vi "CRYLimit Curves Name Replace.vi"(6 "StepName":string, 7 "Setup in":T1={"No.VI"=0, "Category"="", "StepName"="", "Seq setup flattened"="", "Comment"="", "Steps config."=[], "Jump config"=[], "Start"=0.0, "Increment"=0.0, "Name"="Pa", "Unit"="Pa", "Y data"=1, "Y prefix"="", "Y dB ref"=1.0, "Y unit"="", "Repeat State Array"=[]} {"Repeat State Array"."Start" format="%#_5g"; "Y dB ref" format="%.1f"; "Y data" items=["dB", "Lin"]; "Start" format="%#_5g"}, 8 "Hardware Setup In":string, 9 "Step Set up In":string, 11 "Type In":string) -> (3 "Inserted Names Out":string[](array[string]))   [LabVIEW 2013]
uses:
  Typedef Control/CRYStep.ctl
  Typedef Control/CRYData Cluster.ctl
  Typedef Control/CRYWaveform Cluster.ctl
  Typedef Control/CRYResult Cluster.ctl
  CRYMainGlobal.vi
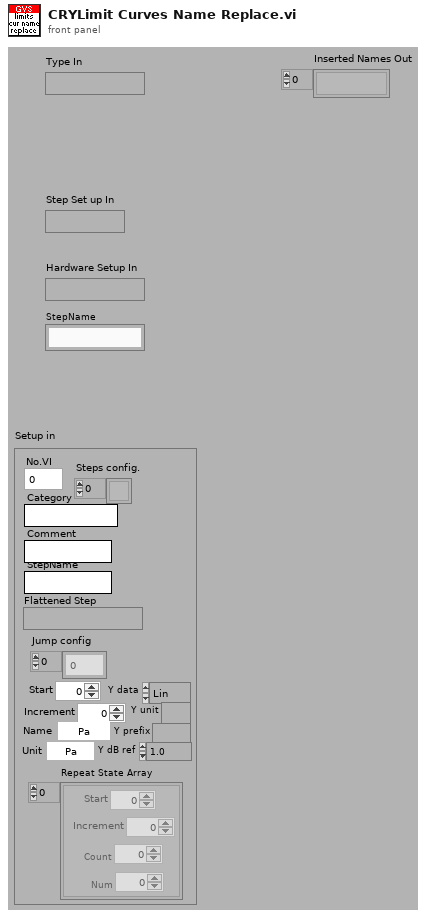
[diagram p1: front panel]
types:
  T1 = typedef "CRYStep.ctl" = cluster{"No.VI":i32, "Category":string, "StepName":string, "Seq setup flattened":string, "Comment":string, "Steps config.":bool[], "Jump config":i32[], "Start":dbl, "Increment":dbl, "Name":string, "Unit":string, "Y data":u16, "Y prefix":string, "Y dB ref":dbl, "Y unit":string, "Repeat State Array":cluster{"Start":dbl, "Increment":dbl, "Count":i32, "Num":i32}[]}
  T2 = typedef "CRYResult Cluster.ctl" = cluster{"Name":string, "Margin":dbl, "unit":string, "Verdict":bool, "Limit":string, "Max/Min":string, "protected":bool, "Step No.":i32, "Test Info":string, "AutoProtect":bool}
  T3 = typedef "CRYWaveform Cluster.ctl" = cluster{"Waveform":cluster{"X0":dbl, "dX":dbl, "Y":sgl[]}, "X data":u16, "Y data":u16, "Y axis":u16, "X unit":string, "Y unit":string, "Y dB ref":dbl, "display Y":bool, "display X":bool, "Overload?":bool, "Test Info":string, "Step No.":i32, "Name":string, "protected":bool, "Sqc history":string[], "Signal Channel ID":i32, "Plot Settings":cluster{"Color":u32, "Interpolation":u8, "Point Style":u8, "Line Style":u8, "Point Color":u32, "Line Width":u8, "Bar Plot Style":u8, "Fill To":i16}, "AutoProtect":bool}
  T4 = typedef "CRYData Cluster.ctl" = cluster{"Name":string, "Curve":cluster{"x":dbl, "y":dbl, "z":dbl}[], "X data":u16, "Y data":u16, "Z data":u16, "X axis":u16, "Y axis":u16, "Z axis":u16, "X unit":string, "Y unit":string, "Z unit":string, "X dB ref":dbl, "Y dB ref":dbl, "Z dB ref":dbl, "single val":bool, "protected":bool, "display X":bool, "display Y":bool, "display Z":bool, "Test Info":string, "Step No.":i32, "Plot Settings":cluster{"Color":u32, "Interpolation":u8, "Point Style":u8, "Line Style":u8, "Point Color":u32, "Line Width":u8, "Bar Plot Style":u8, "Fill To":i16}, "AutoProtect":bool}
  T5 = typedef "CRYLimits.ctl" = cluster{"Name":string, "Tolerance":u16, "X Axis":u16, "Limits":u16, "Upper Limit":cluster{dbl, dbl}[], "Align Ref":cluster{dbl, dbl}, "Lower Limit":cluster{dbl, dbl}[], "Y data":u16, "Y unit":string, "Y dB ref":dbl, "Curve Names":string[], "Y-Resolution":u8, "Type":u16, "x float":bool, "X min-max-step":cluster{"Limit X Offset Min":dbl, "Limit X Offset Max":dbl, "Limit X Offset Step Size":dbl}, "magn/phase":u16, "Upper Limit Type":u16, "Lower Limit Type":u16, "Lim Curve axis up":u16, "Lim Curve axis lo":u16, "Data Selection Upper":u16, "Data Selection Lower":u16, "X-Resolution":u8, "Output failed point curves?":bool, "X data":u16, "X unit":string, "X dB ref":dbl, "X-Y Graph Set-up":string, "Tab Value":enum32{"Data", "Parameters"}, "Help":string, "X Up Val":dbl, "Y Up Val":dbl, "X Low Val":dbl, "Y Low Val":dbl, "Up Limit Val":dbl, "Low Limit Val":dbl, "bAdd DataName":bool, "Custom Name":string}
  T6 = cluster{"Start":dbl, "Increment":dbl, "Count":i32, "Num":i32}[]
  T7 = enum32{"English", "Chinese", "Korean", "Japanese", "Russian", "Chinese traditional"}
  T8 = typedef "CRYData Cluster Array.ctl" = T4[]
  T9 = typedef "CRYWaveform Cluster Array.ctl" = T3[]
  T10 = typedef "CRYResult Cluster Array.ctl" = T2[]
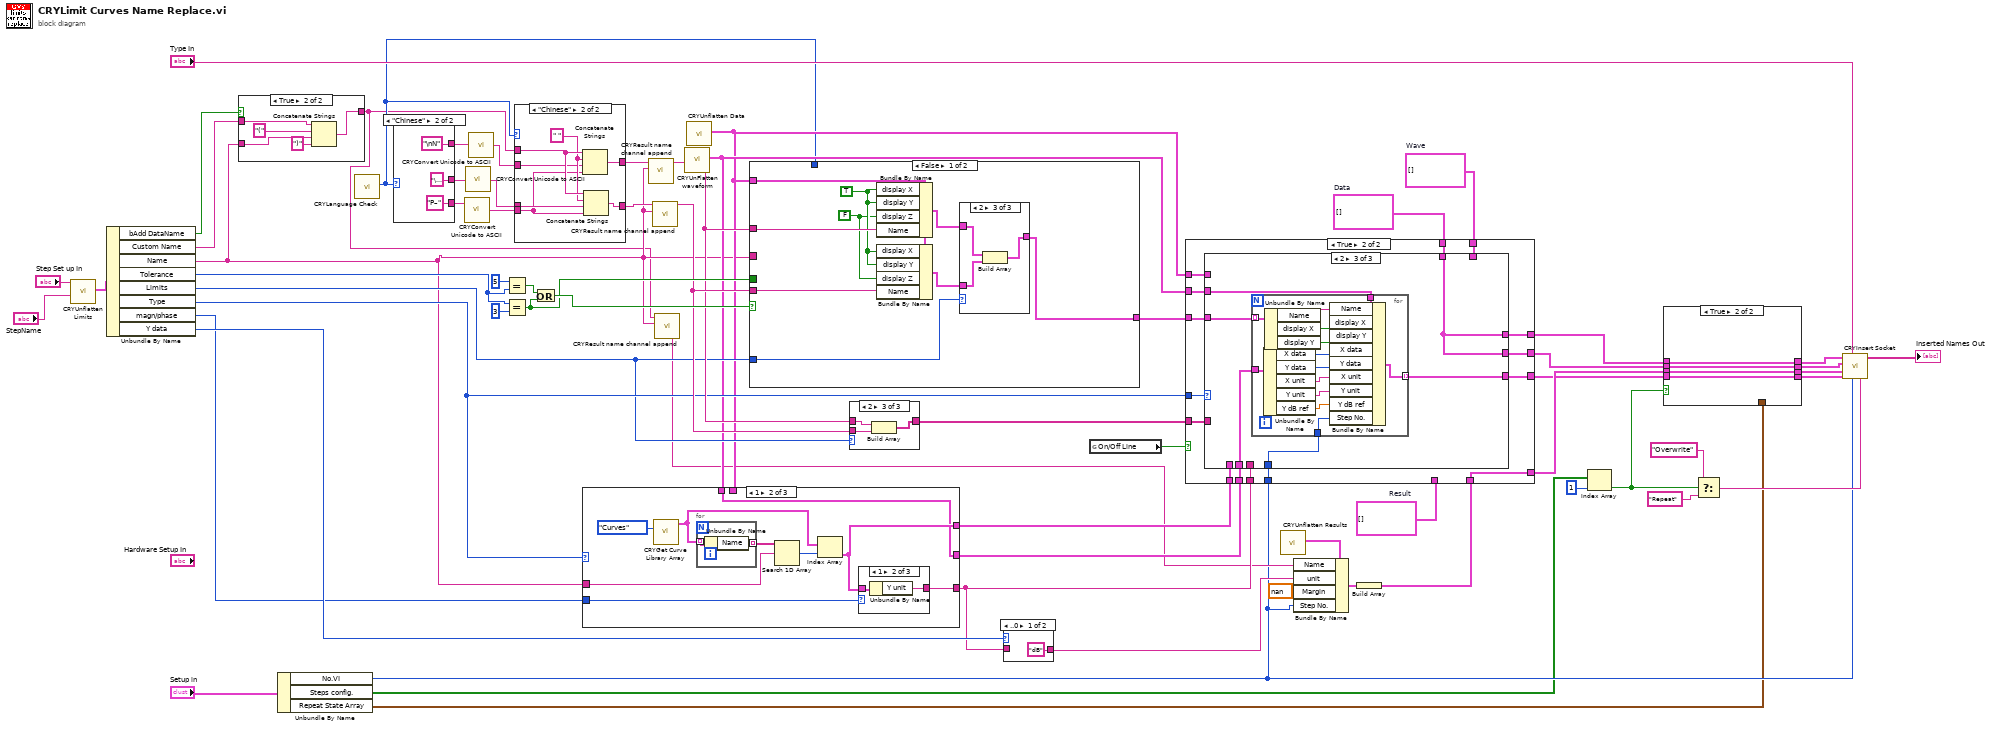
[diagram p0: block diagram]
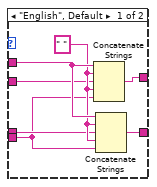
[diagram p3: hidden frame]
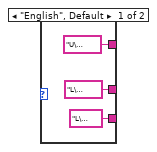
[diagram p4: hidden frame]
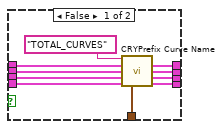
[diagram p5: hidden frame]
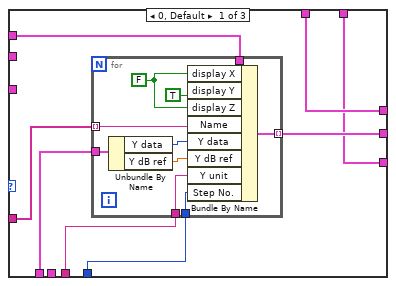
[diagram p7: hidden frame]
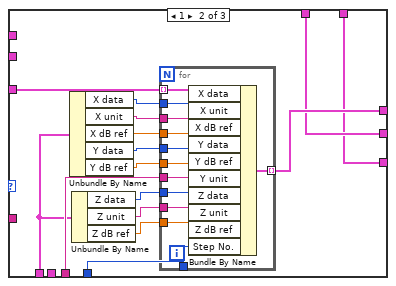
[diagram p8: hidden frame]
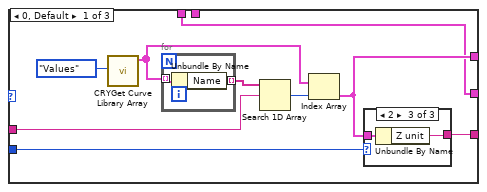
[diagram p9: hidden frame]
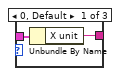
[diagram p10: hidden frame]
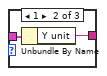
[diagram p11: hidden frame]
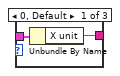
[diagram p12: hidden frame]
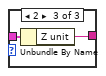
[diagram p13: hidden frame]
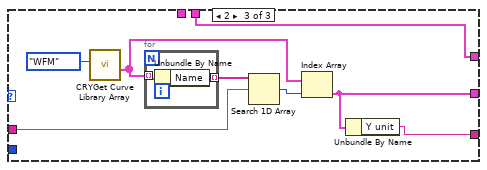
[diagram p14: hidden frame]
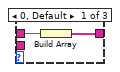
[diagram p16: hidden frame]
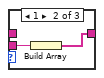
[diagram p17: hidden frame]
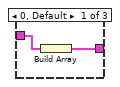
[diagram p18: hidden frame]
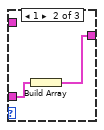
[diagram p19: hidden frame]
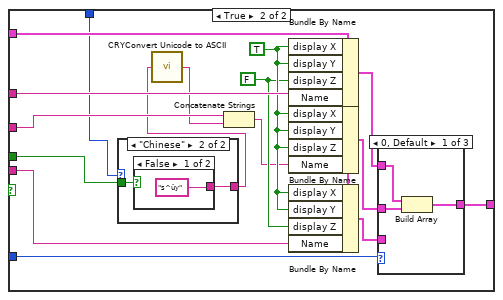
[diagram p20: hidden frame]
diagram:
  w31 = T2[] []  # Result
  w34 = T3[] []  # Wave
  w35 = T4[] []  # Data
  n1 = call "CRYUnflatten Limits.vi"("Step Name"="StepName", "Unflatten Limits"="Step Set up In") -> ("Limits"=w45:T5)  [unwired: 7 in, 2 out]
  n2 = Unbundle By Name(w45) -> ("bAdd DataName"=w5:bool, "Custom Name"=w4:string, "Name"=w3:string, "Tolerance"=w58:u16, "Limits"=w39:u16, "Type"=w44:u16, "magn/phase"=w43:u16, "Y data"=w52:u16)
  n3 = case shown="True" w5 {
    tunnel: w4 -> [w65 w70]
    tunnel: w3 -> [_ w68]
    tunnel: [w65 w66] -> w2
    frame False {
    }
    frame True {
      n4 = Concatenate Strings(w70, "(" ("string"), w68, ")" ("string")) -> (w66:string)
    }
  }
  n5 = Unbundle By Name("Setup in") -> ("No.VI"=w24:i32, "Steps config."=w23:bool[], "Repeat State Array"=w13:T6)
  n6 = call "CRYLanguage Check.vi"() -> ("Language"=w6:T7)  [unwired: 10 in, 1 out]
  n7 = case shown="\"Chinese\"" w6 {
    tunnel: ["L\u0000o\u0000w\u0000e\u0000r\u0000" ("Name") "\u000bN" ("Name")] -> w12
    tunnel: ["L\u0000i\u0000m\u0000i\u0000t\u0000" ("Name") "P–" ("Name")] -> w11
    tunnel: ["U\u0000p\u0000p\u0000e\u0000r\u0000" ("Name") "\nN" ("Name")] -> w10
    frame "English", Default {
    }
    frame "Chinese" {
    }
  }
  n8 = call "CRYConvert Unicode to ASCII.vi"("Unicode"=w11) -> ("ASCII"=w7:string)  [unwired: 4 in]
  n9 = call "CRYConvert Unicode to ASCII.vi"("Unicode"=w12) -> ("ASCII"=w8:string)  [unwired: 4 in]
  n10 = call "CRYConvert Unicode to ASCII.vi"("Unicode"=w10) -> ("ASCII"=w9:string)  [unwired: 4 in]
  n11 = Equal?(x=u16 5, y=w58) -> (x = y?=w59:bool)
  n12 = Equal?(x=w58, y=u16 3) -> (x = y?=w56:bool)
  n13 = case shown="\"Chinese\"" w6 {
    tunnel: [w83 w90] -> w63
    tunnel: [w82 w89] -> w62
    tunnel: w2 -> [w81 w88]
    tunnel: w9 -> [w79 w86]
    tunnel: w8 -> [w78 w85]
    tunnel: w7 -> [w77 w84]
    frame "English", Default {
      w80 = " " ("Name")
      n14 = Concatenate Strings(w81, w80, w79, w80, w77) -> (w83:string)
      n15 = Concatenate Strings(w81, w80, w78, w80, w77) -> (w82:string)
    }
    frame "Chinese" {
      w87 = " " ("Name")
      n16 = Concatenate Strings(w88, w87, w86, w84) -> (w90:string)
      n17 = Concatenate Strings(w88, w87, w85, w84) -> (w89:string)
    }
  }
  n18 = Or(x=w59, y=w56) -> (x .or. y?=w57:bool)
  n19 = call "CRYResult name channel append.vi"("Curve selected"=w3, "Limit step name (no ext.)"=w63) -> ("Result name with channel suffix"=w49:string)  [unwired: 9 out]
  n20 = call "CRYResult name channel append.vi"("Curve selected"=w3, "Limit step name (no ext.)"=w62) -> ("Result name with channel suffix"=w55:string)  [unwired: 9 out]
  n21 = call "CRYResult name channel append.vi"("Curve selected"=w3, "Limit step name (no ext.)"=w2) -> ("Result name with channel suffix"=w30:string)  [unwired: 9 out]
  n22 = call "CRYUnFlatten waveform.vi"() -> ("Waveform Cluster"=w38:T3)  [unwired: 9 in, 2 out]
  n23 = call "CRYUnflatten Data.vi"() -> ("Datum"=w37:T4)  [unwired: 9 in, 2 out]
  n24 = case shown="1" w44 {
    tunnel: w3 -> [w97 w114 w130]
    tunnel: [w94 w110 w125] -> w41
    tunnel: w43 -> [w93 w111 _]
    tunnel: [w92 w109 w127] -> w42
    tunnel: [w91 w108 w126] -> w40
    tunnel: w38 -> [w91 w108 _]
    tunnel: w37 -> [_ _ w125]
    frame 0, Default {
      n25 = call "CRYGet Curve Library Array.vi"("Type In"=enum16{"Curves", "Values", "Results", "WFM"}."Values" ("Type")) -> ("Curve/Value array"=w95:T8)  [unwired: 10 out]
      n26 = for {
        tunnel: w95 -> [w107] mode=indexing
        tunnel: [w106] -> w98 mode=indexing
        n27 = Unbundle By Name(w107) -> ("Name"=w106:string)
      }
      n28 = Search 1D Array(1D array=w98, element=w97) -> (index of element=w96:i32)  [unwired: 1 in]
      n29 = Index Array(array=w95, index=w96) -> (element=w94:T4)
      n30 = case shown="2" w93 {
        tunnel: w94 -> [w101 w103 w105]
        tunnel: [w100 w102 w104] -> w92
        frame 0, Default {
          n31 = Unbundle By Name(w101) -> ("X unit"=w100:string)
        }
        frame 1 {
          n32 = Unbundle By Name(w103) -> ("Y unit"=w102:string)
        }
        frame 2 {
          n33 = Unbundle By Name(w105) -> ("Z unit"=w104:string)
        }
      }
    }
    frame 1 {
      n34 = call "CRYGet Curve Library Array.vi"("Type In"=enum16{"Curves", "Values", "Results", "WFM"}."Curves" ("Type")) -> ("Curve/Value array"=w112:T8)  [unwired: 10 out]
      n35 = for {
        tunnel: w112 -> [w124] mode=indexing
        tunnel: [w123] -> w115 mode=indexing
        n36 = Unbundle By Name(w124) -> ("Name"=w123:string)
      }
      n37 = Search 1D Array(1D array=w115, element=w114) -> (index of element=w113:i32)  [unwired: 1 in]
      n38 = Index Array(array=w112, index=w113) -> (element=w110:T4)
      n39 = case shown="1" w111 {
        tunnel: w110 -> [w118 w120 w122]
        tunnel: [w117 w119 w121] -> w109
        frame 0, Default {
          n40 = Unbundle By Name(w118) -> ("X unit"=w117:string)
        }
        frame 1 {
          n41 = Unbundle By Name(w120) -> ("Y unit"=w119:string)
        }
        frame 2 {
          n42 = Unbundle By Name(w122) -> ("Z unit"=w121:string)
        }
      }
    }
    frame 2 {
      n43 = call "CRYGet Curve Library Array.vi"("Type In"=enum16{"Curves", "Values", "Results", "WFM"}."WFM" ("Type")) -> ("Waveform Array"=w128:T9)  [unwired: 10 out]
      n44 = for {
        tunnel: w128 -> [w134] mode=indexing
        tunnel: [w133] -> w131 mode=indexing
        n45 = Unbundle By Name(w134) -> ("Name"=w133:string)
      }
      n46 = Search 1D Array(1D array=w131, element=w130) -> (index of element=w129:i32)  [unwired: 1 in]
      n47 = Index Array(array=w128, index=w129) -> (element=w126:T3)
      n48 = Unbundle By Name(w126) -> ("Y unit"=w127:string)
    }
  }
  n49 = case shown="False" w57 {
    tunnel: w56 -> [_ w166]
    tunnel: w49 -> [w141 w164]
    tunnel: w55 -> [w139 w161]
    tunnel: w39 -> [w143 w165]
    tunnel: [w142 w158] -> w53
    tunnel: w37 -> [w140 w160]
    tunnel: w3 -> [_ w155]
    tunnel: w6 -> [_ w151]
    frame False {
      w135 = FALSE ("display Z")
      w136 = TRUE ("display X")
      n50 = Bundle By Name(cluster=w140, "display X"=w136, "display Y"=w136, "display Z"=w135, "Name"=w141) -> (w138:T4)
      n51 = Bundle By Name(cluster=w140, "display X"=w136, "display Y"=w136, "display Z"=w135, "Name"=w139) -> (w137:T4)
      n52 = case shown="2" w143 {
        tunnel: w138 -> [w145 _ w150]
        tunnel: w137 -> [_ w147 w149]
        tunnel: [w144 w146 w148] -> w142
        frame 0, Default {
          n53 = Build Array(w145) -> (w144:T4[])
        }
        frame 1 {
          n54 = Build Array(w147) -> (w146:T4[])
        }
        frame 2 {
          n55 = Build Array(w150, w149) -> (w148:T4[])
        }
      }
    }
    frame True {
      w156 = FALSE ("display Z")
      w157 = TRUE ("display X")
      n56 = case shown="\"Chinese\"" w151 {
        tunnel: w166 -> [w168 w172]
        tunnel: [w167 w171] -> w153
        frame "English", Default {
          n57 = case shown="True" w168 {
            tunnel: [" \u0000A\u0000l\u0000i\u0000g\u0000n\u0000e\u0000d\u0000" " \u0000F\u0000l\u0000o\u0000a\u0000t\u0000e\u0000d\u0000"] -> w167
            frame False {
            }
            frame True {
            }
          }
        }
        frame "Chinese" {
          n58 = case shown="False" w172 {
            tunnel: ["s^ûy" ("Unicode") "nm¨R" ("Unicode")] -> w171
            frame False {
            }
            frame True {
            }
          }
        }
      }
      n59 = call "CRYConvert Unicode to ASCII.vi"("Unicode"=w153) -> ("ASCII"=w152:string)  [unwired: 4 in]
      n60 = Concatenate Strings(w155, w152) -> (w154:string)
      n61 = Bundle By Name(cluster=w160, "display X"=w157, "display Y"=w157, "display Z"=w156, "Name"=w164) -> (w163:T4)
      n62 = Bundle By Name(cluster=w160, "display X"=w157, "display Y"=w157, "display Z"=w157, "Name"=w154) -> (w162:T4)
      n63 = Bundle By Name(cluster=w160, "display X"=w157, "display Y"=w157, "display Z"=w156, "Name"=w161) -> (w159:T4)
      n64 = case shown="0, Default" w165 {
        tunnel: w162 -> [w176 w180 w184]
        tunnel: w163 -> [w177 _ w183]
        tunnel: w159 -> [_ w179 w182]
        tunnel: [w175 w178 w181] -> w158
        frame 0, Default {
          n65 = Build Array(w177, w176) -> (w175:T4[])
        }
        frame 1 {
          n66 = Build Array(w180, w179) -> (w178:T4[])
        }
        frame 2 {
          n67 = Build Array(w183, w184, w182) -> (w181:T4[])
        }
      }
    }
  }
  n68 = case shown="2" w39 {
    tunnel: w49 -> [w186 _ w191]
    tunnel: w55 -> [_ w188 w190]
    tunnel: [w185 w187 w189] -> w54
    frame 0, Default {
      n69 = Build Array(w186) -> (w185:string[])
    }
    frame 1 {
      n70 = Build Array(w188) -> (w187:string[])
    }
    frame 2 {
      n71 = Build Array(w191, w190) -> (w189:string[])
    }
  }
  n72 = case shown="..0" w52 {
    tunnel: ["dB" w193] -> w50
    tunnel: w42 -> [_ w193]
    frame ..0 {
    }
    frame 1.. {
    }
  }
  n73 = global read "CRYMainGlobal.vi" "On/Off Line"() -> (w33:bool)
  n74 = call "CRYUnflatten Results.vi"() -> ("Result"=w51:T2)  [unwired: 1 in, 10 out]
  n75 = Bundle By Name(cluster=w51, "Name"=w30, "unit"=w50, "Margin"=nan, "Step No."=w24) -> (w36:T2)
  n76 = Build Array(w36) -> (w32:T2[])
  n77 = case shown="True" w33 {
    tunnel: w54 -> [_ w211]
    tunnel: w53 -> [_ w210]
    tunnel: [w194 w209] -> w21
    tunnel: [w194 w208] -> w22
    tunnel: [w195 w207] -> w19
    tunnel: w24 -> [_ w206]
    tunnel: w44 -> [_ w205]
    tunnel: w42 -> [_ w204]
    tunnel: w41 -> [_ w203]
    tunnel: w40 -> [_ w202]
    tunnel: w38 -> [_ w201]
    tunnel: w37 -> [_ w200]
    tunnel: w35 -> [w194 w199]
    tunnel: w34 -> [w195 w198]
    tunnel: w32 -> [_ w197]
    tunnel: [w196 w197] -> w20
    tunnel: w31 -> [w196 _]
    frame False {
    }
    frame True {
      n78 = case shown="2" w205 {
        tunnel: w211 -> [w219 _ _]
        tunnel: w210 -> [_ w244 w262]
        tunnel: w204 -> [w217 w238 _]
        tunnel: w200 -> [w218 _ _]
        tunnel: w203 -> [w214 w232 _]
        tunnel: w201 -> [_ _ w261]
        tunnel: [w216 w231 w257] -> w209
        tunnel: [w212 w230 w260] -> w207
        tunnel: [w213 w234 w257] -> w208
        tunnel: w206 -> [w215 w233 w259]
        tunnel: w202 -> [_ _ w258]
        tunnel: w199 -> [w213 w231 w257]
        tunnel: w198 -> [w212 w230 _]
        frame 0, Default {
          n79 = for {
            tunnel: w219 -> [w229] mode=indexing
            tunnel: w218 -> [w228]
            tunnel: w214 -> [w227]
            tunnel: w217 -> [w224]
            tunnel: [w220] -> w216 mode=indexing
            tunnel: w215 -> [w221]
            w223 = FALSE ("display X")
            n80 = Unbundle By Name(w227) -> ("Y data"=w226:u16, "Y dB ref"=w225:dbl)
            n81 = Bundle By Name(cluster=w228, "display X"=w223, "display Y"=TRUE, "display Z"=w223, "Name"=w229, "Y data"=w226, "Y dB ref"=w225, "Y unit"=w224, "Step No."=w221) -> (w220:T4)
          }
        }
        frame 1 {
          n82 = Unbundle By Name(w232) -> ("X data"=w243:u16, "X unit"=w242:string, "X dB ref"=w241:dbl, "Y data"=w240:u16, "Y dB ref"=w239:dbl)
          n83 = Unbundle By Name(w232) -> ("Z data"=w237:u16, "Z unit"=w236:string, "Z dB ref"=w235:dbl)
          n84 = for {
            tunnel: w244 -> [w256] mode=indexing
            tunnel: w243 -> [w255]
            tunnel: w242 -> [w254]
            tunnel: w241 -> [w253]
            tunnel: w240 -> [w252]
            tunnel: w239 -> [w251]
            tunnel: w238 -> [w250]
            tunnel: w237 -> [w249]
            tunnel: w236 -> [w248]
            tunnel: w235 -> [w247]
            tunnel: [w245] -> w234 mode=indexing
            tunnel: w233 -> [w246]
            n85 = Bundle By Name(cluster=w256, "X data"=w255, "X unit"=w254, "X dB ref"=w253, "Y data"=w252, "Y dB ref"=w251, "Y unit"=w250, "Z data"=w249, "Z unit"=w248, "Z dB ref"=w247, "Step No."=w246) -> (w245:T4)
          }
        }
        frame 2 {
          n86 = for {
            tunnel: w262 -> [w274] mode=indexing
            tunnel: w261 -> [w275]
            tunnel: w258 -> [w270]
            tunnel: [w263] -> w260 mode=indexing
            tunnel: w259 -> [w264]
            n87 = Unbundle By Name(w270) -> ("X data"=w269:u16, "Y data"=w268:u16, "X unit"=w267:string, "Y unit"=w266:string, "Y dB ref"=w265:dbl)
            n88 = Unbundle By Name(w274) -> ("Name"=w273:string, "display X"=w272:bool, "display Y"=w271:bool)
            n89 = Bundle By Name(cluster=w275, "Name"=w273, "display X"=w272, "display Y"=w271, "X data"=w269, "Y data"=w268, "X unit"=w267, "Y unit"=w266, "Y dB ref"=w265, "Step No."=w264) -> (w263:T3)
          }
        }
      }
    }
  }
  n90 = Index Array(array=w23, index=1) -> (element=w14:bool)
  n91 = case shown="True" w14 {
    tunnel: w22 -> [w285 w289]
    tunnel: w21 -> [w284 w288]
    tunnel: w20 -> [w283 w287]
    tunnel: w19 -> [w282 w286]
    tunnel: [w281 w286] -> w18
    tunnel: [w280 w287] -> w17
    tunnel: [w279 w288] -> w16
    tunnel: [w278 w289] -> w15
    tunnel: w13 -> [w276 _]
    frame False {
      n92 = call "CRYPrefix Curve Name.vi"("Type In"="TOTAL_CURVES", "Curves In"=w285, "Values In"=w284, "Results In"=w283, "Waves In"=w282, "Repeat State Array In"=w276) -> ("Curves Out"=w278:T8, "Values Out"=w279:T8, "Results Out"=w280:T10, "Waves Out"=w281:T9)  [unwired: 6 in]
    }
    frame True {
    }
  }
  n93 = Select(t="Overwrite" ("Y unit"), s=w14, f="Repeat") -> (s? t:f=w26:string)
  n94 = call "CRYInsert Socket.vi"("sOption2"=w26, "Step No."=w24, "sOption1"="Type In", "Waves"=w18, "Results"=w17, "Values"=w16, "Curves"=w15) -> ("Inserted Names Out"=→"Inserted Names Out":string[])  [unwired: 4 in]
